vi "Read String.vi"(8 "error in (no error)":errorcluster, 11 "Subset_STR in":refnum<class "Insert_STR.lvclass">) -> (0 "error out":errorcluster, 2 "Abs_String.lvclass":refnum<class "Abs_String.lvclass">, 3 "Subset_STR out":refnum<class "Insert_STR.lvclass">)   [LabVIEW 2021, in "Insert_STR.lvclass"]
uses:
  Insert_STR.lvclass
  Abs_Types/String/Abs_String.lvclass
  Insert_STR.lvclass/Insert_STR.ctl
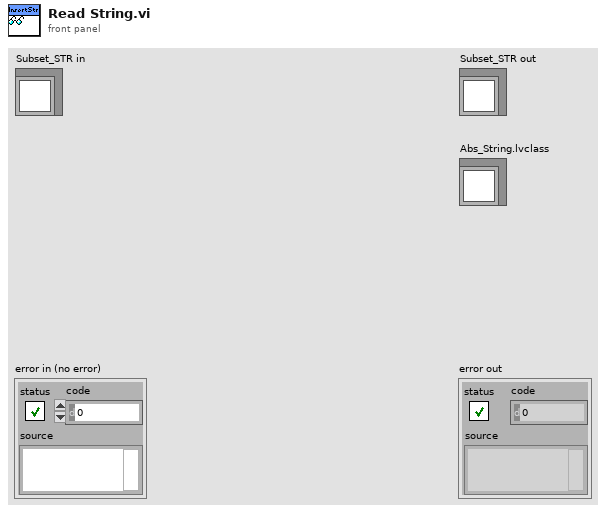
[diagram p1: front panel]
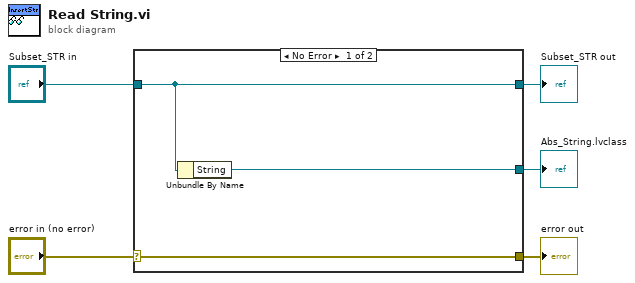
[diagram p0: block diagram]
diagram:
  n1 = case shown="No Error" "error in (no error)" {
    selector: "error in (no error)" -> [w8 w9]
    tunnel: [w8 w9] -> w4
    tunnel: [w7 w10] -> w2
    tunnel: "Subset_STR in" -> [w7 w10]
    tunnel: [w6 _] -> w1
    frame No Error {
      n2 = Unbundle By Name(w7) -> ("String"=w6:refnum<class "Abs_String.lvclass">)
    }
    frame Error {
    }
  }
  "error out" <- w4
  "Subset_STR out" <- w2
  "Abs_String.lvclass" <- w1
